vi "OCR.vi"() -> ()   [LabVIEW 2021]
uses:
  <vilib>/vision/NI_Vision_Development_Module.lvlib
panel:
  in  "Character Index":dbl
  out "Character Value 2":string
  out "Read String":string
  in  "정지":bool
  in  "판별":bool
  in  "Character Value":string
  in  "학습파일확인":bool
  in  "저장":bool
  in  "학습":bool
  in  "File Path":path
  out "Image":T1(plugin-control)
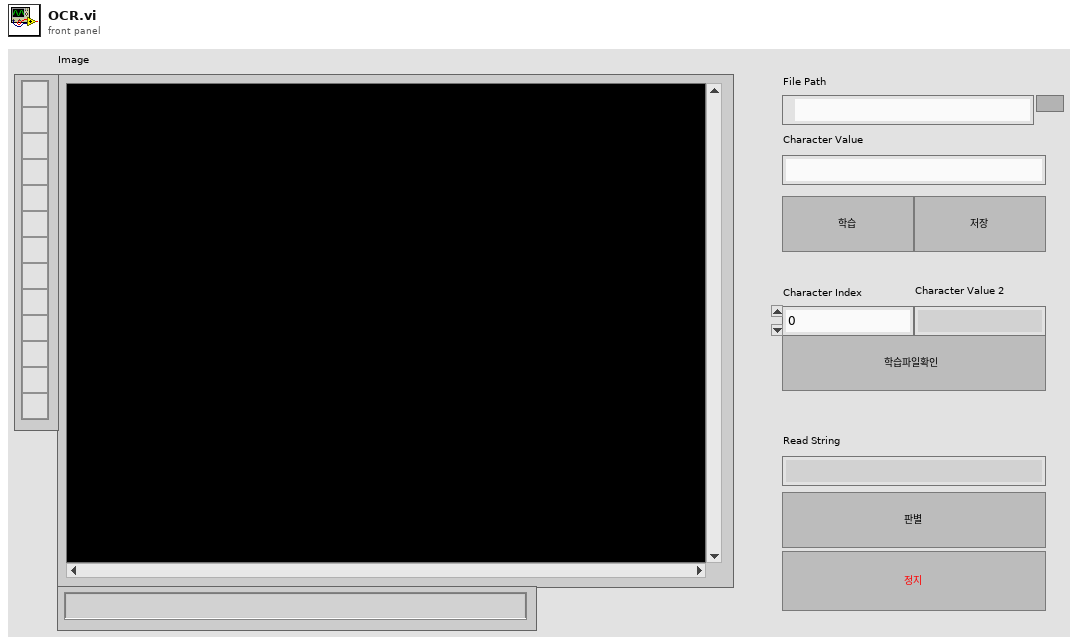
[diagram p1: front panel]
types:
  T1 = typedef "IMAQ Image.ctl" = refnum<image>
  T2 = typedef "Image Type" = u32
  T3 = typedef "ROI Descriptor" = cluster{"Global Rectangle":i32[], "Contours":cluster{"ID":enum32{"External", "Internal"}, "Type":u32, "Coordinates":i32[]}[]}
  T4 = cluster{"샘플파일":path, "학습파일":path, "ROI Descriptor Out":T3}
  T5 = typedef "IMAQ OCR Session.ctl" = refnum<k1>
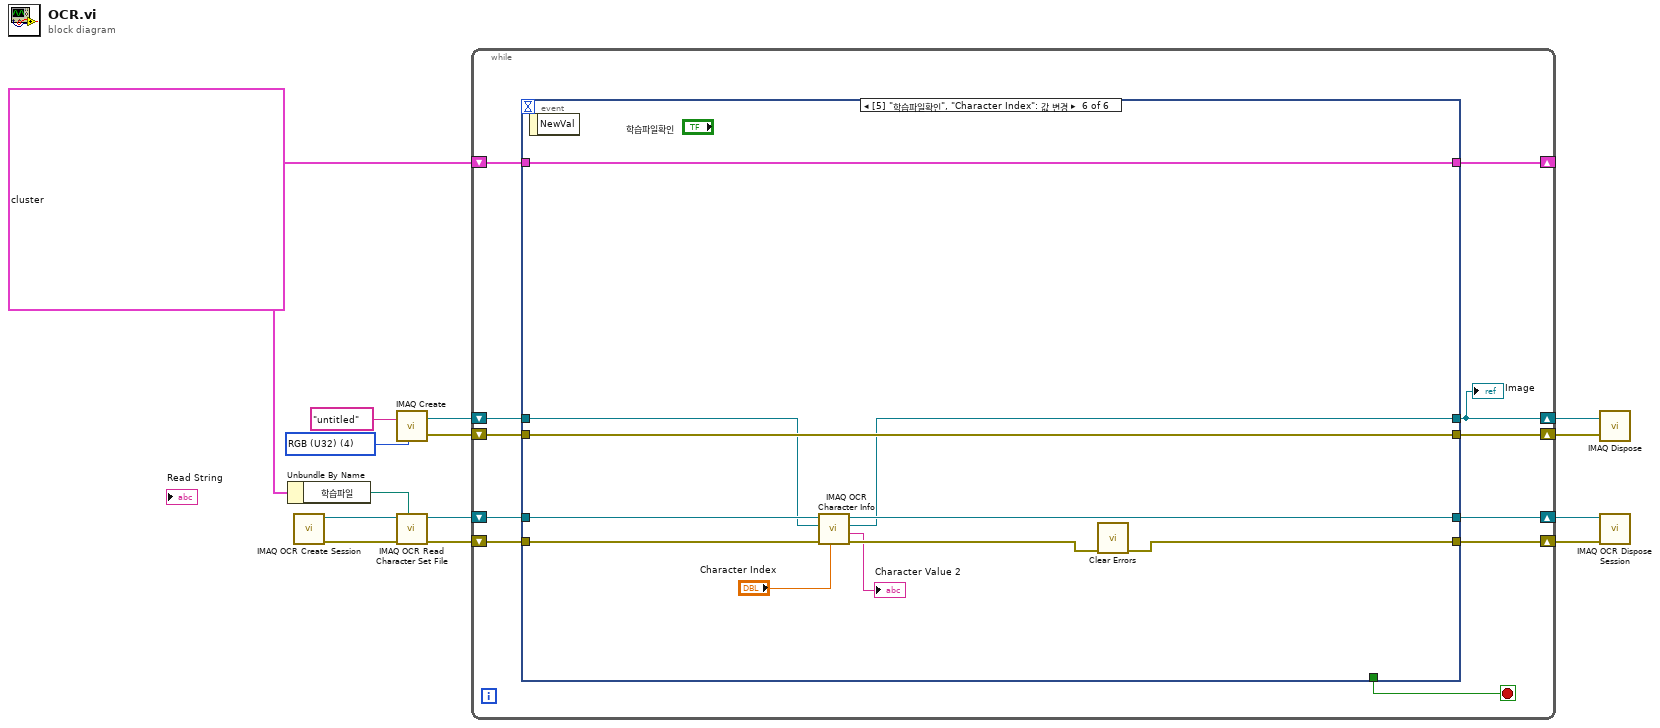
[diagram p0: block diagram]
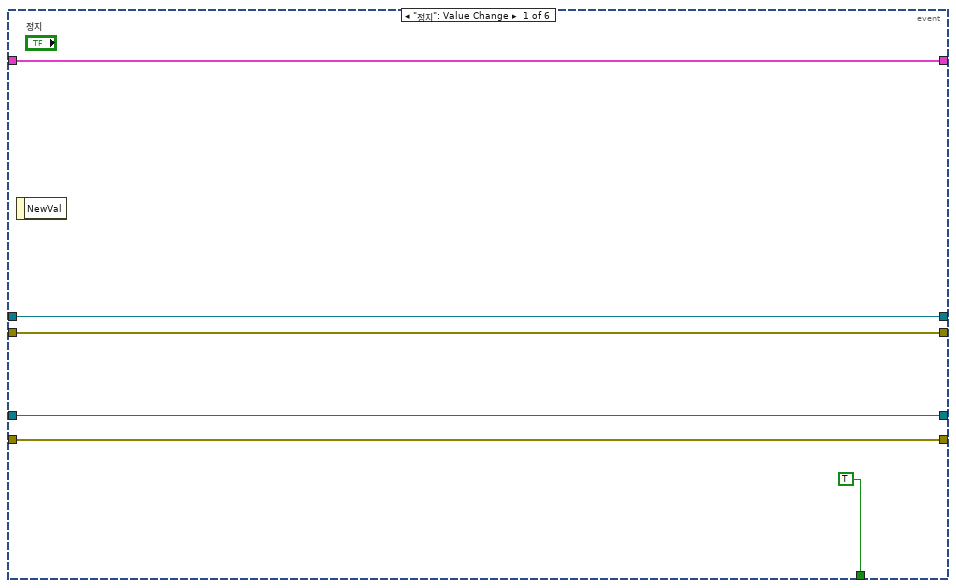
[diagram p2: hidden frame]
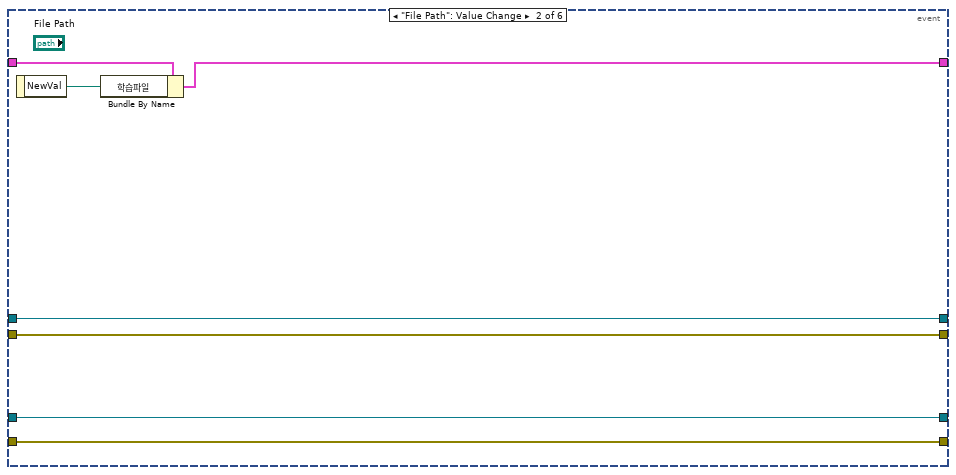
[diagram p3: hidden frame]
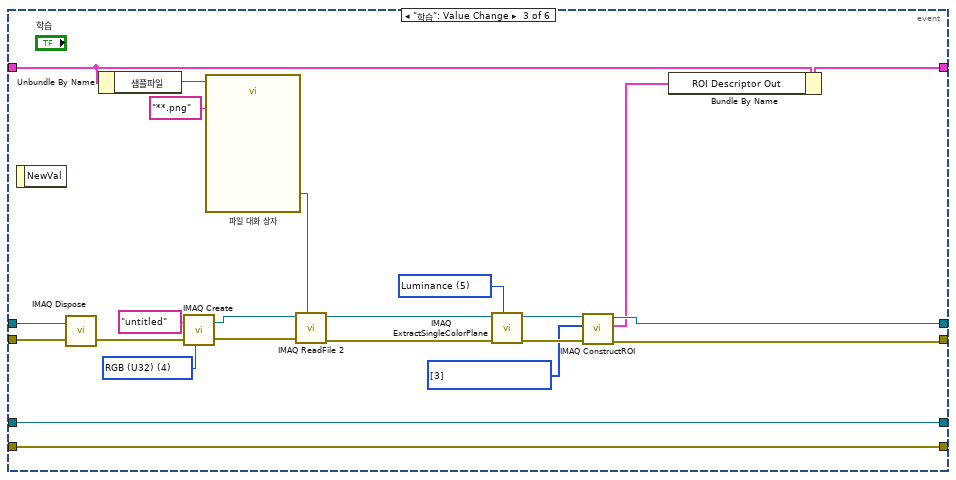
[diagram p4: hidden frame]
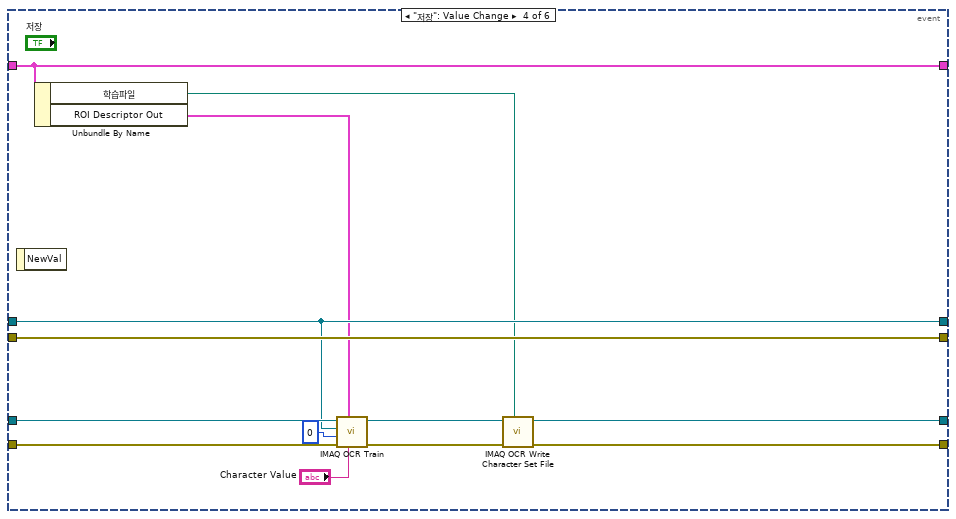
[diagram p5: hidden frame]
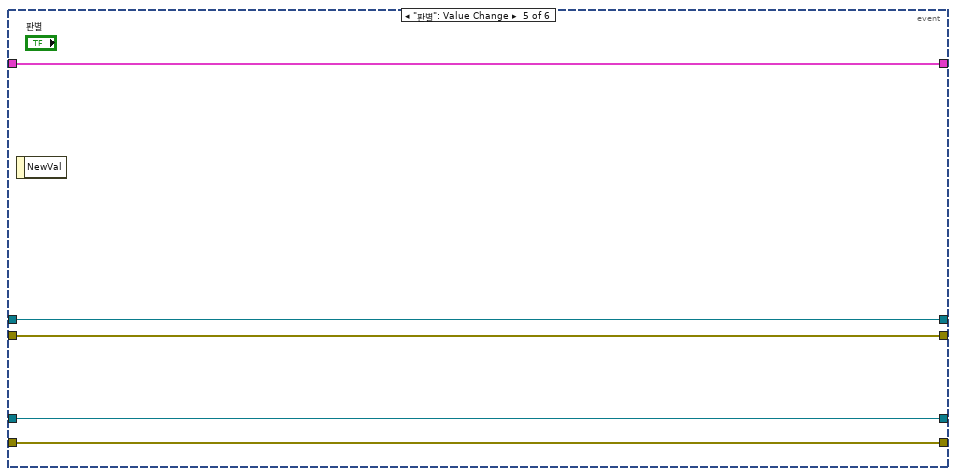
[diagram p6: hidden frame]
diagram:
  w13 = T2 4 items=["Grayscale (U8)", "Grayscale (I16)", "Grayscale (SGL)", "Complex (CSG)", "RGB (U32)", "HSL (U32)", "RGB (U64)", "Grayscale (U16)"] ("Image Type")
  w6 = T4 {"샘플파일"=path "C:/Embedded_System/04_LabVIEW/Programming_SourceCode/LabVIEW/이미지파일/OCR", "학습파일"=path "C:/Embedded_System/04_LabVIEW/Programming_SourceCode/LabVIEW/이미지파일/OCR/학습.abc", "ROI Descriptor Out"={"Global Rectangle"=[], "Contours"=[]}}
  n1 = Unbundle By Name(w6) -> ("학습파일"=w5:path)
  n2 = call "IMAQ OCR Create Session"() -> ("error out"=w7:errorcluster, "IMAQ OCR Session"=w8:T5)  [unwired: 10 in]
  n3 = call "IMAQ Create"("Image Name"="untitled", "Image Type"=w13) -> ("New Image"=w12:T1, "error out"=w11:errorcluster)  [unwired: 3 in]
  n4 = call "IMAQ OCR Read Character Set File"("File Path"=w5, "error in (no error)"=w7, "IMAQ OCR Session"=w8) -> ("error out"=w9:errorcluster, "IMAQ OCR Session (dup)"=w10:T5)  [unwired: 6 in, 1 out]
  n5 = while {
    shift-right: [w25] -> _
    shift-left: w6 -> [w24]
    shift-right: [w15] -> w4
    shift-left: w12 -> [w22]
    shift-right: [w18] -> w2
    shift-left: w10 -> [w21]
    shift-right: [w17] -> w1
    shift-left: w9 -> [w19]
    shift-right: [w16] -> w3
    shift-left: w11 -> [w23]
    stop <- w20 stop-if-true
    n6 = event shown="[5] \"학습파일확인\", \"Character Index\": 값 변경" {
      selector: _ -> [_ _ _ _ _ _]
      dyn-events: _ -> [_ _ _ _ _ _]
      timeout: _ -> [_ _ _ _ _ _]
      tunnel: [w31 w34 w39 w73 w79 w90] -> w25
      tunnel: w24 -> [w31 w35 w41 w73 w79 w90]
      tunnel: w23 -> [w26 w33 w56 w74 w75 w89]
      tunnel: [w30 w38 w43 w70 w78 w80] -> w15
      tunnel: w22 -> [w30 w38 w57 w70 w78 w81]
      tunnel: w21 -> [w29 w37 w61 w72 w77 w88]
      tunnel: [w29 w37 w61 w67 w77 w86] -> w18
      tunnel: [TRUE _ _ _ _ _] -> w20
      tunnel: [w27 w36 w60 w66 w76 w84] -> w17
      tunnel: w19 -> [w27 w36 w60 w71 w76 w87]
      tunnel: [w26 w33 w42 w74 w75 w89] -> w16
      event "정지": Value Change {
        n7 = event-data() -> ()  [unwired: 1 in, 1 out]
      }
      event "File Path": Value Change {
        n8 = event-data() -> ("NewVal"=w32:path)  [unwired: 1 in]
        n9 = Bundle By Name(cluster=w35, "학습파일"=w32) -> (w34:T4)
      }
      event "학습": Value Change {
        w44 = T2 4 items=["Grayscale (U8)", "Grayscale (I16)", "Grayscale (SGL)", "Complex (CSG)", "RGB (U32)", "HSL (U32)", "RGB (U64)", "Grayscale (U16)"] ("Image Type")
        w47 = 5 items=["Red", "Green", "Blue", "Hue", "Saturation", "Luminance", "Value", "Intensity"] ("Color Plane")
        w48 = u32[] [3] items=["No Selection", "Point", "Line", "Rectangle", "Oval", "Polygon", "Freehand Region", "Annulus", "Zoom", "Pan", "Broken Line", "Freehand Line", "Rotated Rectangle"] ("Tools")
        n10 = event-data() -> ()  [unwired: 1 in, 1 out]
        n11 = call "IMAQ Dispose"("Image"=w57, "error in (no error)"=w56) -> ("error out"=w55:errorcluster)  [unwired: 4 in]
        n12 = Unbundle By Name(w41) -> ("샘플파일"=w59:path)
        n13 = call "IMAQ Create"("Image Name"="untitled", "Image Type"=w44, "error in (no error)"=w55) -> ("New Image"=w51:T1, "error out"=w54:errorcluster)  [unwired: 2 in]
        n14 = call "파일 대화 상자"("start path"=w59, "pattern (all files)"="**.png") -> ("selected path"=w46:path)  [unwired: 10 in, 3 out]
        n15 = call "IMAQ ReadFile 2"("File Path"=w46, "error in (no error)"=w54, "Image"=w51) -> ("error out"=w53:errorcluster, "Image Out"=w50:T1)  [unwired: 4 in, 3 out]
        n16 = call "IMAQ ExtractSingleColorPlane"("Color Plane"=w47, "error in (no error)"=w53, "Image Src"=w50) -> ("error out"=w52:errorcluster, "Image Dst Out"=w49:T1)  [unwired: 1 in, 6 out]
        n17 = call "IMAQ ConstructROI"("error in (no error)"=w52, "Tools"=w48, "Image"=w49) -> ("error out"=w42:errorcluster, "ROI Descriptor Out"=w40:T3, "Image Out (duplicate)"=w43:T1)  [unwired: 5 in, 1 out]
        n18 = Bundle By Name(cluster=w41, "ROI Descriptor Out"=w40) -> (w39:T4)
      }
      event "저장": Value Change {
        n19 = event-data() -> ()  [unwired: 1 in, 1 out]
        n20 = Unbundle By Name(w73) -> ("학습파일"=w68:path, "ROI Descriptor Out"=w69:T3)
        n21 = call "IMAQ OCR Train"("Character Value"="Character Value", "ROI Descriptor"=w69, "error in (no error)"=w71, "Object Index"=0, "Image"=w70, "IMAQ OCR Session"=w72) -> ("error out"=w64:errorcluster, "IMAQ OCR Session (dup)"=w65:T5)  [unwired: 3 in, 1 out]
        n22 = call "IMAQ OCR Write Character Set File"("File Path"=w68, "error in (no error)"=w64, "IMAQ OCR Session"=w65) -> ("error out"=w66:errorcluster, "IMAQ OCR Session (dup)"=w67:T5)  [unwired: 7 in]
      }
      event "판별": Value Change {
        n23 = event-data() -> ()  [unwired: 1 in, 1 out]
      }
      event "학습파일확인", "Character Index": Value Change {
        n24 = event-data() -> ()  [unwired: 1 in, 1 out]
        n25 = call "IMAQ OCR Character Info"("Character Index"="Character Index", "error in (no error)"=w87, "Character Image"=w81, "IMAQ OCR Session"=w88) -> ("error out"=w85:errorcluster, "Character Value"=→"Character Value 2":string, "Character Image (out)"=w80:T1, "IMAQ OCR Session (dup)"=w86:T5)  [unwired: 2 in, 2 out]
        n26 = call <vilib>:"Clear Errors.vi"("error in (no error)"=w85) -> ("error out"=w84:errorcluster)  [unwired: 5 in, 1 out]
      }
    }
    "Image" <- w15
  }
  n27 = call "IMAQ Dispose"("Image"=w4, "error in (no error)"=w3) -> ()  [unwired: 4 in, 1 out]
  n28 = call "IMAQ OCR Dispose Session"("error in (no error)"=w1, "IMAQ OCR Session"=w2) -> ()  [unwired: 9 in, 1 out]
